vi "EPTx FPGA-SquIn.vi"() -> ()   [LabVIEW 2019]
uses:
  <vilib>/Powertrain Controls/Device Drivers/Engine Position Tracking/EPTx/RevA/FPGA/Controls/EPTxSupervisor.ctl
  <vilib>/Powertrain Controls/Device Drivers/Engine Position Tracking/EPTx/RevA/FPGA/Controls/EPTxTooth.ctl
  <vilib>/Powertrain Controls/Device Drivers/Engine Position Tracking/EPTx/RevA/FPGA/Controls/EPTxConfig.ctl
  <vilib>/Powertrain Controls/Device Drivers/Engine Position Tracking/EPTx/RevA/FPGA/Controls/EPTxControl.ctl
  <vilib>/Powertrain Controls/Device Drivers/Engine Position Tracking/EPTx/RevA/FPGA/Controls/EPTxSignals.ctl
  <vilib>/Powertrain Controls/Device Drivers/Engine Position Tracking/EPTx/RevA/FPGA/Controls/EPTxAAPControl.ctl
  <vilib>/Powertrain Controls/Device Drivers/Engine Position Tracking/EPTx/RevA/FPGA/Controls/EPTxSimulatorConfig.ctl
  <vilib>/Powertrain Controls/Device Drivers/Engine Position Tracking/EPTx/RevA/FPGA/Controls/EPTxPatternConfig.ctl
  <vilib>/Powertrain Controls/Device Drivers/Engine Position Tracking/EPTx/RevA/FPGA/Controls/Patterns.ctl
  <vilib>/Powertrain Controls/Device Drivers/Engine Position Tracking/EPTx/RevA/FPGA/Controls/EPTxDebug.ctl
  <vilib>/Platform/TimedLoop/XDataNode/timing_clust.ctl
  <vilib>/Platform/TimedLoop/XDataNode/nitl_modes.ctl
  <vilib>/Platform/TimedLoop/XDataNode/wakeup.ctl
  <vilib>/rvi/Emulation/niFpgaSctlEmulationGetInTimedLoop.vi
  <vilib>/rvi/Emulation/niFpgaEmulationReportErrorSimple.vi
  <vilib>/rvi/Emulation/niFpgaGetClockAttributes.vi
  <vilib>/rvi/Emulation/niFpgaCriticalErrorInLSC.vi
  <vilib>/rvi/eio/common/nirviEmuTemplateMethod_errors.vi
  <vilib>/Platform/TimedLoop/XDataNode/XDataNode.xnode
  <vilib>/eio/EIONode/EIONode.xnode
  <vilib>/Platform/TimedLoop/XDataNode/XDNodeRunTimeDep.lvlib
  <vilib>/Powertrain Controls/Device Drivers/Engine Position Tracking/EPTx/RevA/FPGA/EPTx - RevA - FPGA.lvlib
panel:
  in  "当前转速":fxp<+,24,14>
  out "PatternOutput":T1
  out "EPTxDebug":T2
  in  "EPTxPatternConfig":T3 {"Pattern"."Aux 4" format="%#_16g"; "Pattern"."Aux 3" format="%#_16g"; "Pattern"."Aux 2" format="%#_16g"; "Pattern"."Aux 1" format="%#_16g"; "Pattern"."Primary" format="%#_16g"}
  in  "EPTxSimulatorConfig":T5
  in  "CamSim_AAPControl":T6
  out "EPTxSignals":T1
  in  "EPTxControl":T7
  in  "EPTxConfig":T8
  out "EPTxTooth":T9
  out "EPTxSupervisor":T10
  out "Loop":u32
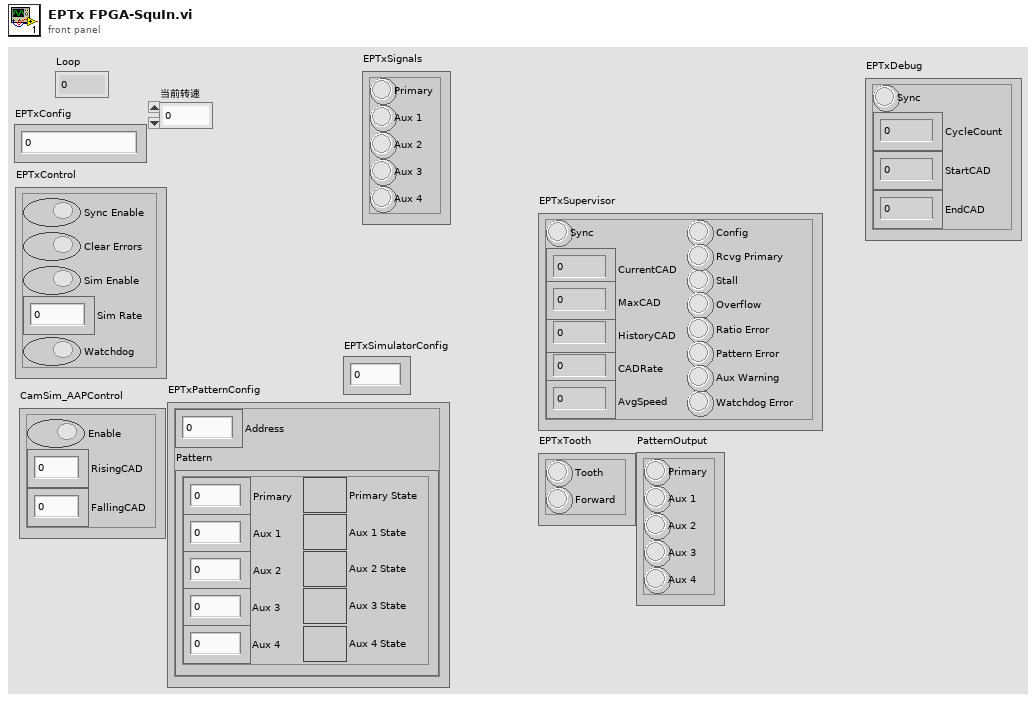
[diagram p1: front panel]
types:
  T1 = typedef "EPTx - RevA - FPGA.lvlib/EPTxSignals.ctl" = cluster{"Primary":bool, "Aux 1":bool, "Aux 2":bool, "Aux 3":bool, "Aux 4":bool}
  T2 = typedef "EPTx - RevA - FPGA.lvlib/EPTxDebug.ctl" = cluster{"Sync":bool, "CycleCount":fxp<+,8,8>, "StartCAD":fxp<+,18,11>, "EndCAD":fxp<+,18,11>}
  T3 = typedef "EPTx - RevA - FPGA.lvlib/EPTxPatternConfig.ctl" = cluster{"Address":fxp<+,14,14>, "Pattern":T4}
  T4 = typedef "EPTx - RevA - FPGA.lvlib/Patterns.ctl" = cluster{"Primary":fxp<+,19,12>, "Primary State":bool, "Aux 1":fxp<+,19,12>, "Aux 1 State":bool, "Aux 2":fxp<+,19,12>, "Aux 2 State":bool, "Aux 3":fxp<+,19,12>, "Aux 3 State":bool, "Aux 4":fxp<+,19,12>, "Aux 4 State":bool}
  T5 = typedef "EPTx - RevA - FPGA.lvlib/EPTxSimulatorConfig.ctl" = u32
  T6 = typedef "EPTx - RevA - FPGA.lvlib/EPTxAAPControl.ctl" = cluster{"Enable":bool, "RisingCAD":fxp<+,18,11>, "FallingCAD":fxp<+,18,11>}
  T7 = typedef "EPTx - RevA - FPGA.lvlib/EPTxControl.ctl" = cluster{"Sync Enable":bool, "Clear Errors":bool, "Sim Enable":bool, "Sim Rate":fxp<+,24,6>, "Watchdog":bool}
  T8 = typedef "EPTx - RevA - FPGA.lvlib/EPTxConfig.ctl" = u64
  T9 = typedef "EPTx - RevA - FPGA.lvlib/EPTxTooth.ctl" = cluster{"Tooth":bool, "Forward":bool}
  T10 = typedef "EPTx - RevA - FPGA.lvlib/EPTxSupervisor.ctl" = cluster{"Sync":bool, "CurrentCAD":fxp<+,18,11>, "MaxCAD":fxp<+,11,11>, "HistoryCAD":fxp<+,11,11>, "CADRate":fxp<+,22,8>, "AvgSpeed":fxp<+,17,15>, "Config":bool, "Rcvg Primary":bool, "Stall":bool, "Overflow":bool, "Ratio Error":bool, "Pattern Error":bool, "Aux Warning":bool, "Watchdog Error":bool}
  T11 = typedef "XDNodeRunTimeDep.lvlib/timing_clust.ctl" = cluster{"Expected End [f-1]":u64, "Actual End [f-1]":u64, "Finished Late? [f-1]":bool, "Expected End [i-1]":u64, "Actual End [i-1]":u64, "Finished Late? [i-1]":bool, "Expected Start [i]":u64, "Actual Start [i]":u64, "Expected Start [f]":u64, "Actual Start [f]":u64, "Source Name":string, "Structure Name":string, "Period":i64, "Deadline":i64, "Offset":i64, "Start":i64, "Priority":i32, "Timeout":i32, "Mode":T12, "Wakeup Reason":T13, "Error":errorcluster, "Source Type":string, "Secondary Source Type":string, "Global End Time":u64, "Global Start Time":u64, "Frame Duration":u64, "Iteration Duration":u64, "Assigned CPU":i32, "I/O Scan Engine Mode":u32}
  T12 = typedef "XDNodeRunTimeDep.lvlib/nitl_modes.ctl" = enum32{"No Change", "Process missed periods, maintain original phase", "Discard missed periods, maintain original phase", "Process missed periods, ignore original phase", "Discard missed periods, ignore original phase"}
  T13 = typedef "XDNodeRunTimeDep.lvlib/wakeup.ctl" = enum32{"Normal", "Aborted", "Asynchronous wakeup", "Timing source error", "Timed loop error", "Timeout"}
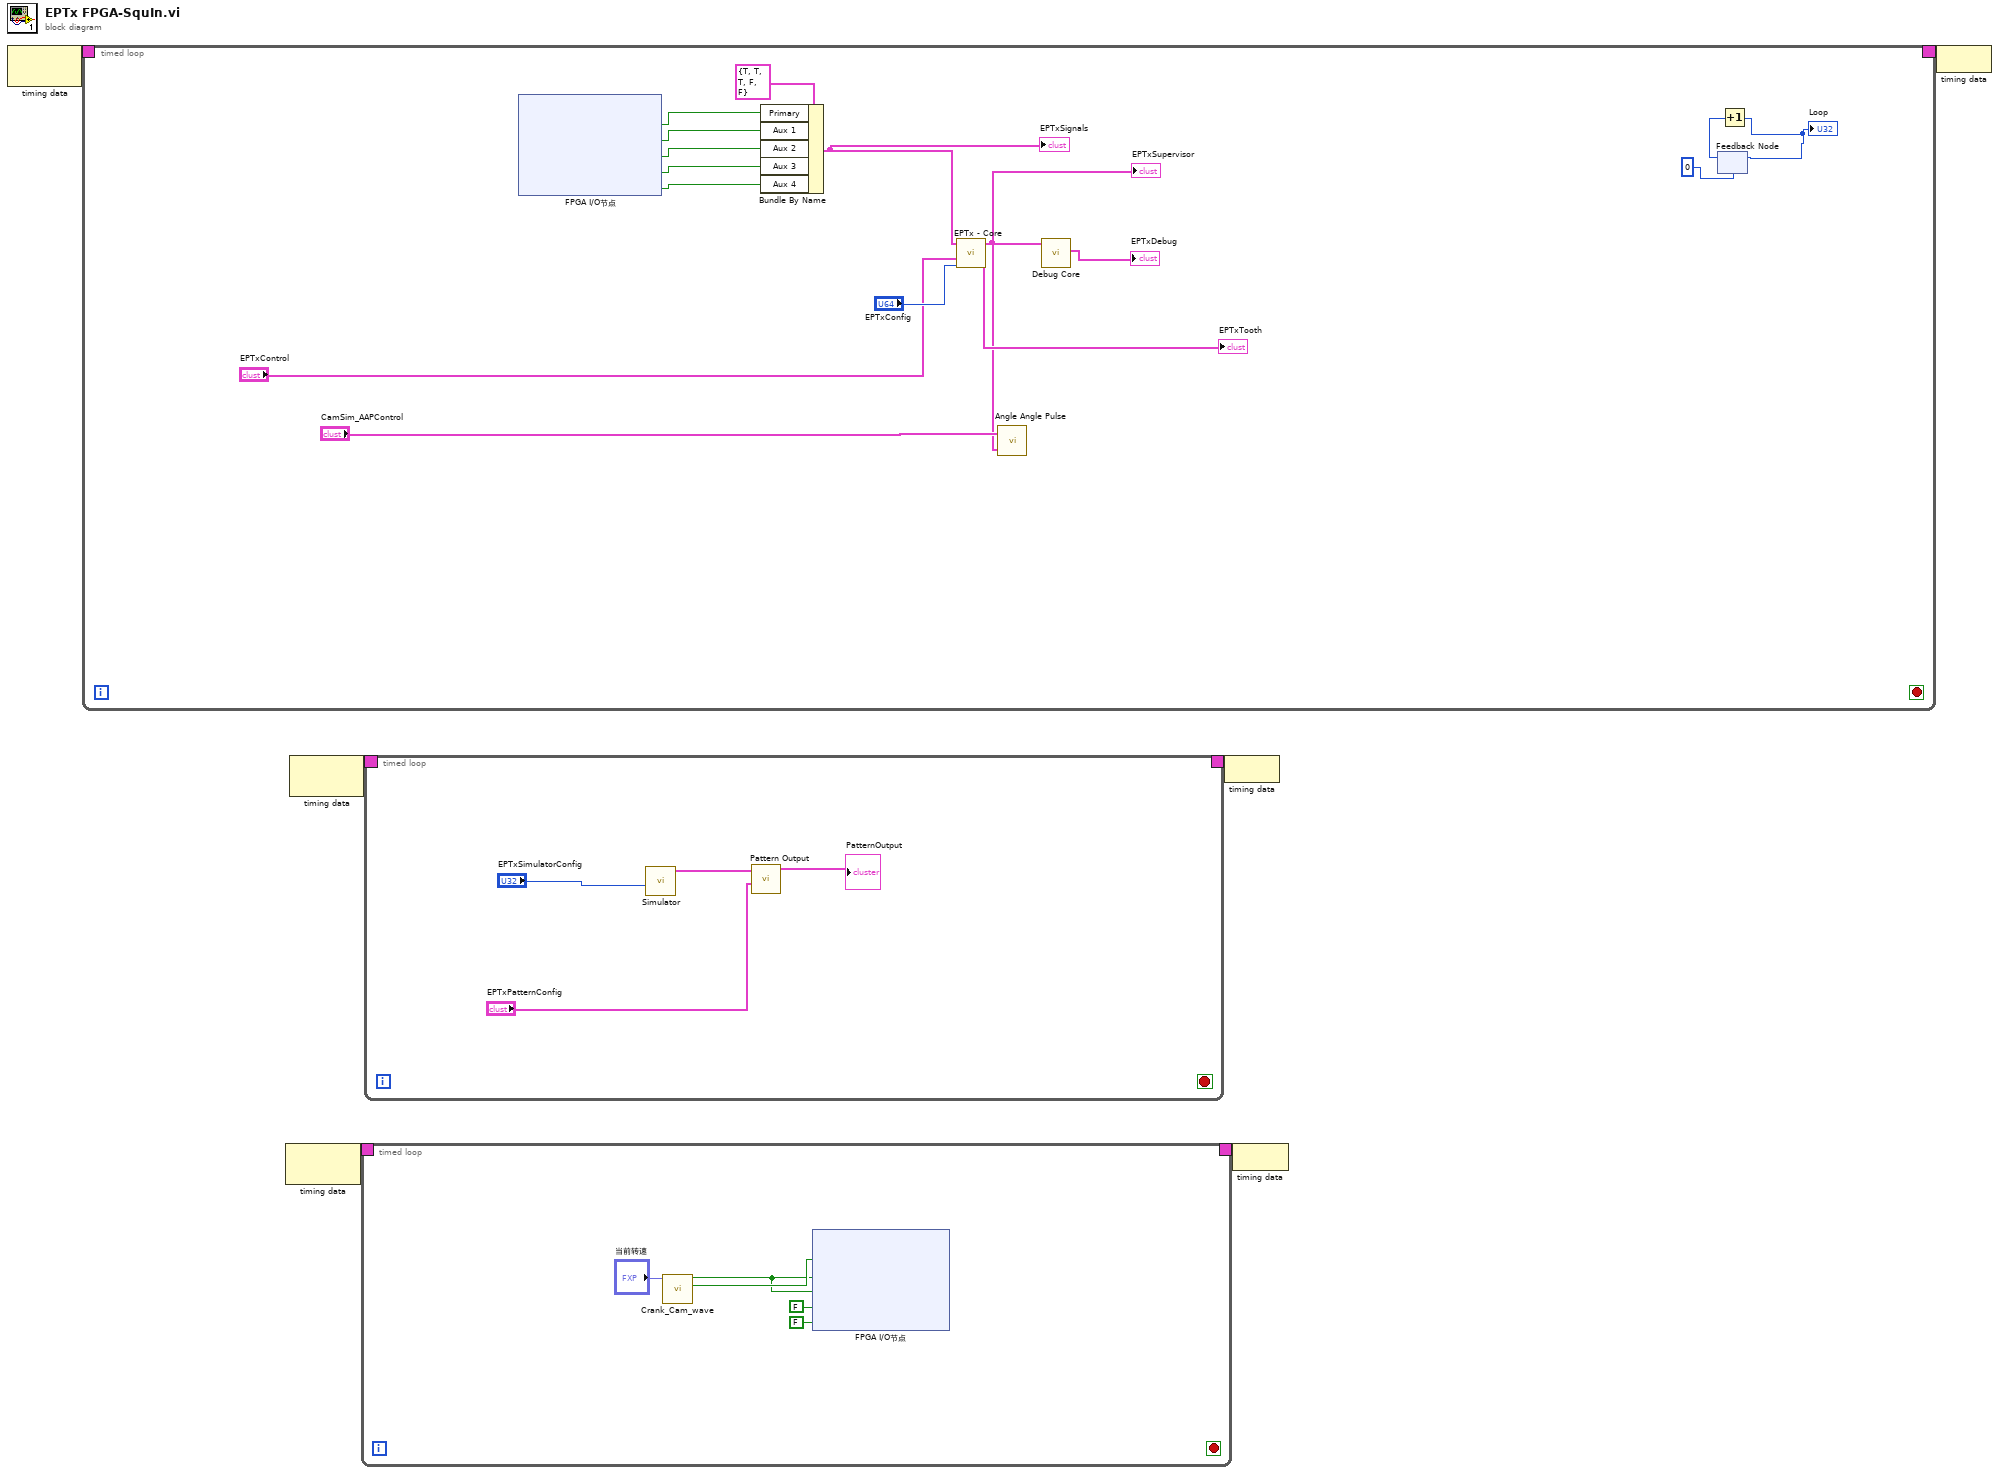
[diagram p0: block diagram]
diagram:
  n1 = node-c288() -> (w6:T11)  [unwired: 1 in]
  n2 = timed-loop {
    timing: w6 -> [_]
    timing-out: [_] -> w5
    stop <- _ stop-if-true
    n3 = xnode "FPGA I/O节点"() -> ("Connector0/DIO8"=w12:bool, "Connector0/DIO9"=w11:bool, "Connector0/DIO10"=w10:bool, "Connector0/DIO11"=w9:bool, "Connector0/DIO12"=w8:bool)  [unwired: 5 in, 5 out]
    n4 = Bundle By Name(cluster=T1 {"Primary"=TRUE, "Aux 1"=TRUE, "Aux 2"=TRUE, "Aux 3"=FALSE, "Aux 4"=FALSE} ("EPTxSignals"), "Primary"=w12, "Aux 1"=w11, "Aux 2"=w10, "Aux 3"=w9, "Aux 4"=w8) -> (w7:T1)
    "EPTxSignals" <- w7
    n5 = call <vilib>:"EPTx - Core.vi"("EPTxConfig"="EPTxConfig", "EPTxControl"="EPTxControl", "EPTxSignals"=w7) -> ("EPTxTooth"=→"EPTxTooth":T9, "EPTxSupervisor"=w16:T10)  [unwired: 7 in]
    "EPTxSupervisor" <- w16
    n6 = call <vilib>:"Angle Angle Pulse.vi"("EPTxSupervisor"=w16, "AAPControl"="CamSim_AAPControl") -> ()  [unwired: 1 out]
    n7 = call <vilib>:"Debug Core.vi"("EPTxSupervisor"=w16) -> ("EPTxDebug"=→"EPTxDebug":T2)  [unwired: 10 in]
    n8 = feedback #1(u32 0) -> (w22:u32)
    n9 = Increment(x=w22) -> (x+1=w21:u32)
    "Loop" <- w21
    n10 = feedback-in #1(w21) -> ()
  }
  n11 = node-c288() -> (w2:T11)  [unwired: 1 in]
  n12 = node-c288() -> (w4:T11)  [unwired: 1 in]
  n13 = timed-loop {
    timing: w2 -> [_]
    timing-out: [_] -> w1
    stop <- _ stop-if-true
    n14 = call "Crank_Cam_wave.vi"("当前转速"="当前转速") -> ("曲轴"=w28:bool, "凸轮轴"=w27:bool)  [unwired: 9 in]
    n15 = xnode "FPGA I/O节点"("Connector0/DIO0"=w28, "Connector0/DIO1"=w27, "Connector0/DIO2"=w27, "Connector0/DIO3"=FALSE, "Connector0/DIO4"=FALSE) -> ()  [unwired: 5 in, 5 out]
  }
  n16 = timed-loop {
    timing: w4 -> [_]
    timing-out: [_] -> w3
    stop <- _ stop-if-true
    n17 = call <vilib>:"Simulator.vi"("EPTxSimulatorConfig"="EPTxSimulatorConfig") -> ("EPTxSupervisor"=w33:T10)  [unwired: 10 in]
    n18 = call <vilib>:"Pattern Output.vi"("EPTxPatternConfig"="EPTxPatternConfig", "EPTxSupervisor"=w33) -> ("PatternOutput"=→"PatternOutput":T1)  [unwired: 9 in]
  }
  n19 = node-c288(w3) -> ()
  n20 = node-c288(w1) -> ()
  n21 = node-c288(w5) -> ()
